vi "FusePose.vi"(0 "Vision Valid [t-?]":bool, 1 "Odometry Timestamp (ms)":u32, 2 "Odometry Delta X (in) [t0]":dbl, 3 "Odometry Delta Y (in) [t0]":dbl, 5 "Vision X (in) [t-?]":dbl, 7 "Vision Y (in) [t-?]":dbl, 9 "Vision Timestamp (ms)":u32, 12 "Pose Mode":T1(ring)) -> (4 "X (in) [t0]":dbl, 6 "Y (in) [t0]":dbl, 10 "X Odometry Only (in) [t0]":dbl, 15 "Y Odometry Only (in) [t0]":dbl)   [LabVIEW 2020]
doc: "This VI fuses multiple sensing modalities to estimate the robot's current pose."
uses:
  <vilib>/Rock Robotics/WPI/DriverStation/WPI_DriverStationRobotMode2.ctl
  7b9bb9b1-306e-4d3e-b7ed-2eba6d8170c6.vi
  1559d662-8abd-40e9-a5dc-3c53134ee71a.vi
  524daecc-998c-4826-9d6e-2db19cf0bc7c.vi
  GlobalDriverStationData.vi
  GlobalDrivebase.vi
  GlobalPoseAndTargeting.vi
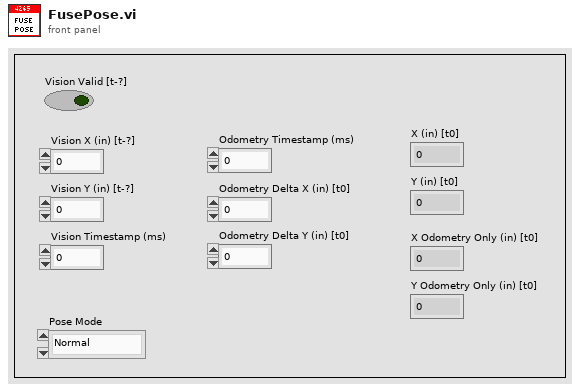
[diagram p1: front panel]
types:
  T1 = enum16{"Normal", "Auto Set", "Reset IMU", "Manual Push", "Init"}
  T2 = typedef "WPI_DriverStationRobotMode2.ctl" = enum16{"Autonomous Disabled", "Autonomous Enabled", "Teleop Disabled", "Teleop Enabled", "Disconnected", "Finish", "Test Disabled", "Test Enabled", "Emergency Stopped"}
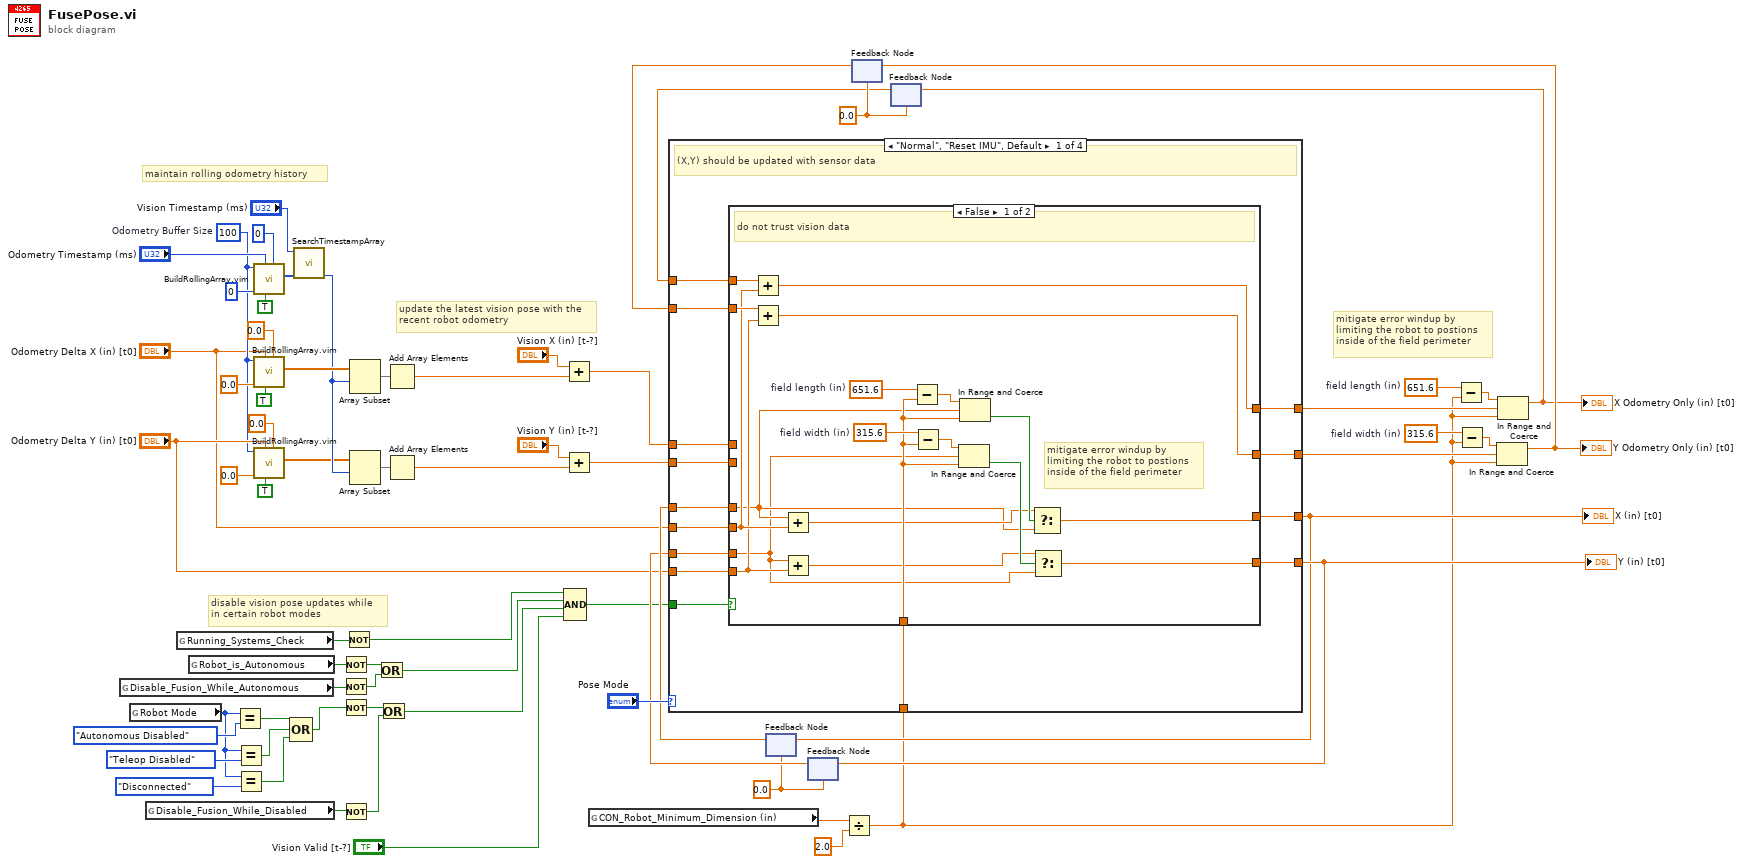
[diagram p0: block diagram]
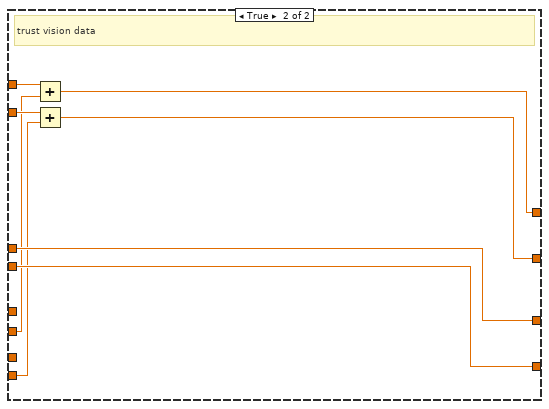
[diagram p2: hidden frame]
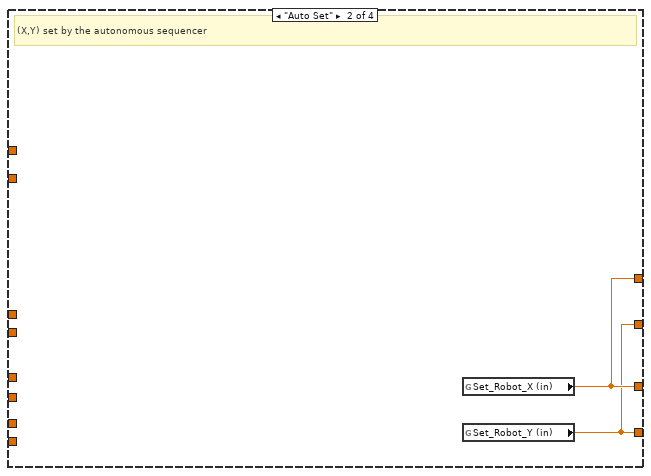
[diagram p3: hidden frame]
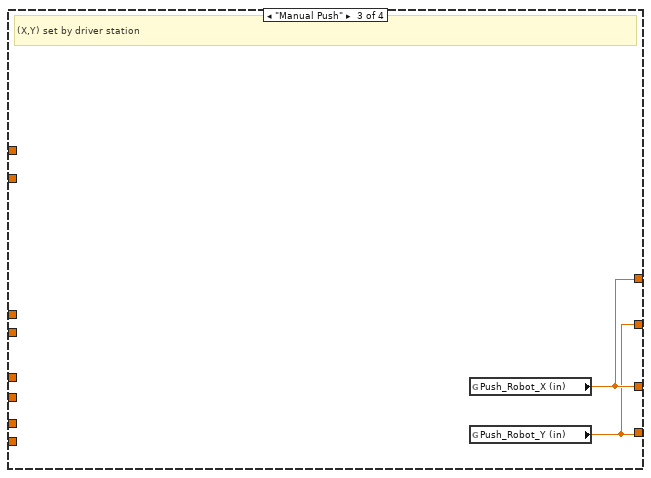
[diagram p4: hidden frame]
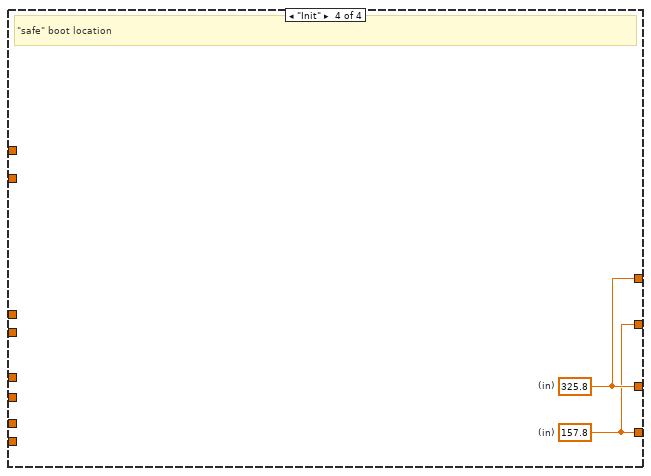
[diagram p5: hidden frame]
diagram:
  w15 = 0.0
  w48 = 0.0
  w17 = 651.6  # field length (in)
  w16 = 315.6  # field width (in)
  w12 = 100  # Odometry Buffer Size
  # "disable vision pose updates while\nin certain robot modes"
  # "maintain rolling odometry history"
  # "update the latest vision pose with the\nrecent robot odometry"
  # "mitigate error windup by\nlimiting the robot to postions\ninside of the field perimeter"
  n1 = global read "GlobalDriverStationData.vi" "Disable_Fusion_While_Autonomous"() -> (w38:bool)
  n2 = global read "GlobalDriverStationData.vi" "Robot Mode"() -> (w27:T2)
  n3 = global read "GlobalDriverStationData.vi" "Disable_Fusion_While_Disabled"() -> (w41:bool)
  n4 = global read "GlobalDriverStationData.vi" "Running_Systems_Check"() -> (w3:bool)
  n5 = global read "GlobalDriverStationData.vi" "Robot_is_Autonomous"() -> (w40:bool)
  n6 = Equal?(x=w27, y=WPI_DriverStationRobotMode2."Autonomous Disabled" ("Robot Mode")) -> (x = y?=w32:bool)
  n7 = Equal?(x=w27, y=WPI_DriverStationRobotMode2."Teleop Disabled") -> (x = y?=w30:bool)
  n8 = Equal?(x=w27, y=WPI_DriverStationRobotMode2."Disconnected") -> (x = y?=w25:bool)
  n9 = call "BuildRollingArray.vim"("Global Additive Update"=0, "Update?"=TRUE, "New Value"="Odometry Timestamp (ms)", "Initial Value"=0, "Number of Elements"=w12) -> ("Current Array"=w63:u32[])  [unwired: 6 in]
  n10 = call "BuildRollingArray.vim"("Global Additive Update"=0.0, "Update?"=TRUE, "New Value"="Odometry Delta X (in) [t0]", "Initial Value"=0.0, "Number of Elements"=w12) -> ("Current Array"=w60:dbl[])  [unwired: 6 in]
  n11 = call "BuildRollingArray.vim"("Global Additive Update"=0.0, "Update?"=TRUE, "New Value"="Odometry Delta Y (in) [t0]", "Initial Value"=0.0, "Number of Elements"=w12) -> ("Current Array"=w55:dbl[])  [unwired: 6 in]
  n12 = Compound Arithmetic op=OR(w32, w30, w25) -> (w31:bool)
  n13 = call "SearchTimestampArray.vi"("Timestamp Array"=w63, "Search Timestamp"="Vision Timestamp (ms)") -> ("Closest Index"=w56:i32)  [unwired: 8 in, 1 out]
  n14 = Not(x=w40) -> (.not. x?=w39:bool)
  n15 = Not(x=w38) -> (.not. x?=w37:bool)
  n16 = Not(x=w31) -> (.not. x?=w34:bool)
  n17 = Not(x=w41) -> (.not. x?=w35:bool)
  n18 = Not(x=w3) -> (.not. x?=w2:bool)
  n19 = Array Subset(array=w60, index=w56) -> (w61:dbl[])  [unwired: 1 in]
  n20 = Array Subset(array=w55, index=w56) -> (w58:dbl[])  [unwired: 1 in]
  n21 = Or(x=w39, y=w37) -> (x .or. y?=w36:bool)
  n22 = Or(x=w34, y=w35) -> (x .or. y?=w33:bool)
  n23 = Add Array Elements(numeric array=w61) -> (sum=w59:dbl)
  n24 = Add Array Elements(numeric array=w58) -> (sum=w57:dbl)
  n25 = Add(x="Vision X (in) [t-?]", y=w59) -> (x+y=w52:dbl)
  n26 = Add(x="Vision Y (in) [t-?]", y=w57) -> (x+y=w53:dbl)
  n27 = Compound Arithmetic op=AND(w2, w36, w33, "Vision Valid [t-?]") -> (w42:bool)
  n28 = global read "GlobalDrivebase.vi" "CON_Robot_Minimum_Dimension (in)"() -> (w1:dbl)
  n29 = feedback #1(w48) -> (w50:dbl)
  n30 = feedback #2(w48) -> (w49:dbl)
  n31 = Divide(x=w1, y=2.0) -> (x/y=w4:dbl)
  n32 = feedback #3(w15) -> (w13:dbl)
  n33 = feedback #4(w15) -> (w14:dbl)
  n34 = case shown="\"Normal\", \"Reset IMU\", Default" "Pose Mode" {
    tunnel: [w77 w110 w112 w114] -> w9
    tunnel: w50 -> [w81 _ _ _]
    tunnel: "Odometry Delta X (in) [t0]" -> [w80 _ _ _]
    tunnel: w49 -> [w79 _ _ _]
    tunnel: "Odometry Delta Y (in) [t0]" -> [w78 _ _ _]
    tunnel: [w76 w109 w111 w113] -> w10
    tunnel: w42 -> [w75 _ _ _]
    tunnel: w53 -> [w74 _ _ _]
    tunnel: w52 -> [w73 _ _ _]
    tunnel: [w72 w110 w112 w114] -> w6
    tunnel: [w71 w109 w111 w113] -> w8
    tunnel: w14 -> [w70 _ _ _]
    tunnel: w13 -> [w69 _ _ _]
    tunnel: w4 -> [w68 _ _ _]
    frame "Normal", "Reset IMU", Default {
      # "(X,Y) should be updated with sensor data"
      n35 = case shown="False" w75 {
        tunnel: w81 -> [w83 _]
        tunnel: w80 -> [w96 w102]
        tunnel: w79 -> [w82 _]
        tunnel: w78 -> [w95 w101]
        tunnel: [w89 w107] -> w77
        tunnel: [w88 w108] -> w76
        tunnel: w74 -> [_ w108]
        tunnel: w73 -> [_ w107]
        tunnel: [w98 w105] -> w72
        tunnel: [w97 w104] -> w71
        tunnel: w70 -> [w100 w106]
        tunnel: w69 -> [w99 w103]
        tunnel: w68 -> [w90 _]
        frame False {
          w92 = 651.6  # field length (in)
          w91 = 315.6  # field width (in)
          # "mitigate error windup by\nlimiting the robot to postions\ninside of the field perimeter"
          # "do not trust vision data"
          n36 = Add(x=w100, y=w96) -> (x+y=w98:dbl)
          n37 = Add(x=w99, y=w95) -> (x+y=w97:dbl)
          n38 = Add(x=w83, y=w96) -> (x+y=w85:dbl)
          n39 = Add(x=w82, y=w95) -> (x+y=w84:dbl)
          n40 = Subtract(x=w92, y=w90) -> (x-y=w94:dbl)
          n41 = Subtract(x=w91, y=w90) -> (x-y=w93:dbl)
          n42 = In Range and Coerce(upper limit=w93, x=w82, lower limit=w90) -> (In Range?=w86:bool)  [unwired: 1 out]
          n43 = In Range and Coerce(upper limit=w94, x=w83, lower limit=w90) -> (In Range?=w87:bool)  [unwired: 1 out]
          n44 = Select(t=w85, s=w87, f=w83) -> (s? t:f=w89:dbl)
          n45 = Select(t=w84, s=w86, f=w82) -> (s? t:f=w88:dbl)
        }
        frame True {
          # "trust vision data"
          n46 = Add(x=w106, y=w102) -> (x+y=w105:dbl)
          n47 = Add(x=w103, y=w101) -> (x+y=w104:dbl)
        }
      }
    }
    frame "Auto Set" {
      # "(X,Y) set by the autonomous sequencer"
      n48 = global read "GlobalPoseAndTargeting.vi" "Set_Robot_X (in)"() -> (w110:dbl)
      n49 = global read "GlobalPoseAndTargeting.vi" "Set_Robot_Y (in)"() -> (w109:dbl)
    }
    frame "Manual Push" {
      # "(X,Y) set by driver station"
      n50 = global read "GlobalPoseAndTargeting.vi" "Push_Robot_X (in)"() -> (w112:dbl)
      n51 = global read "GlobalPoseAndTargeting.vi" "Push_Robot_Y (in)"() -> (w111:dbl)
    }
    frame "Init" {
      w113 = 157.8  # (in)
      w114 = 325.8  # (in)
      # "\"safe\" boot location"
    }
  }
  "X (in) [t0]" <- w9
  "Y (in) [t0]" <- w10
  n52 = feedback-in #1(w9) -> ()
  n53 = feedback-in #2(w10) -> ()
  n54 = Subtract(x=w17, y=w4) -> (x-y=w18:dbl)
  n55 = Subtract(x=w16, y=w4) -> (x-y=w19:dbl)
  n56 = In Range and Coerce(upper limit=w19, x=w8, lower limit=w4) -> (coerced(x)=w7:dbl)  [unwired: 1 out]
  "Y Odometry Only (in) [t0]" <- w7
  n57 = feedback-in #3(w7) -> ()
  n58 = In Range and Coerce(upper limit=w18, x=w6, lower limit=w4) -> (coerced(x)=w5:dbl)  [unwired: 1 out]
  "X Odometry Only (in) [t0]" <- w5
  n59 = feedback-in #4(w5) -> ()
